vi "Construct.vi"(5 "Mailserver":string, 6 "Buffer":u32, 7 "Subject":string, 8 "Error in (no error)":errorcluster, 9 "Recipients":string[](array[string]), 10 "LogFormatterInterface in":refnum<class "LogFormatterInterface.lvclass">) -> (0 "Error out":errorcluster, 3 "LogWriterEmail out":refnum<class "LogWriterEmail.lvclass">)   [LabVIEW 2011, in "LogWriterEmail.lvclass"]
uses:
  LogWriterEmail.lvclass
  Formatter/LogFormatterInterface/LogFormatterInterface.lvclass
  LogWriterEmail.lvclass/LogWriterEmail.ctl
  LogWriterMock/LogWriterMock.lvclass
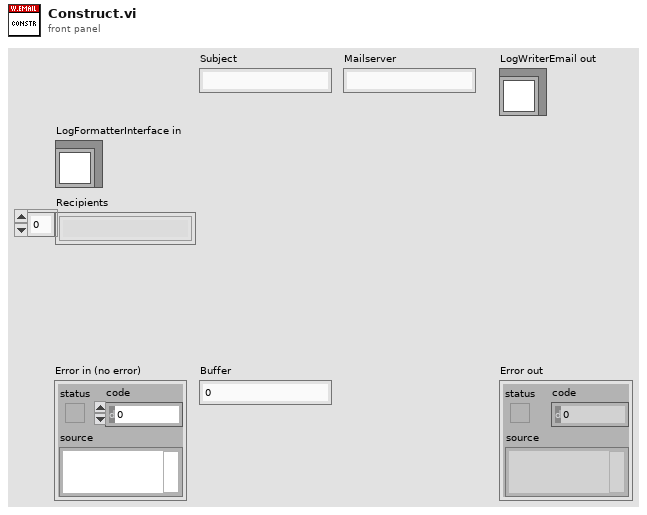
[diagram p1: front panel]
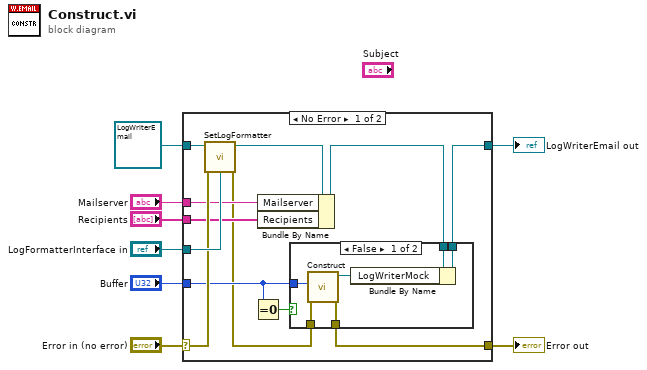
[diagram p0: block diagram]
diagram:
  n1 = case shown="No Error" "Error in (no error)" {
    selector: "Error in (no error)" -> [w18 w30]
    tunnel: [w11 w30] -> w7
    tunnel: [w9 w29] -> w6
    tunnel: refnum<class "LogWriterEmail.lvclass"> refnum ("LogWriterEmail in") -> [w19 w29]
    tunnel: "LogFormatterInterface in" -> [w20 _]
    tunnel: "Mailserver" -> [w16 _]
    tunnel: "Recipients" -> [w15 _]
    tunnel: "Buffer" -> [w13 _]
    frame No Error {
      n2 = call-dynamic "SetLogFormatter.vi"("Error in (no error)"=w18, "LogFormatterInterface in"=w20, "LogWriterEmail in"=w19) -> ("Error out"=w12:errorcluster, "LogWriterEmail out"=w17:refnum<class "LogWriterEmail.lvclass">)  [unwired: 7 in]
      n3 = Equal To 0?(x=w13) -> (x = 0?=w14:bool)
      n4 = Bundle By Name(cluster=w17, "Mailserver"=w16, "Recipients"=w15) -> (w10:refnum<class "LogWriterEmail.lvclass">)
      n5 = case shown="False" w14 {
        tunnel: w13 -> [w26 _]
        tunnel: w10 -> [w22 w28]
        tunnel: w12 -> [w25 w27]
        tunnel: [w24 w27] -> w11
        tunnel: [w21 w28] -> w9
        frame False {
          n6 = call "Construct.vi"("Error in (no error)"=w25, "Buffer"=w26) -> ("Error out"=w24:errorcluster, "LogWriterMock out"=w23:refnum<class "LogWriterMock.lvclass">)  [unwired: 8 in]
          n7 = Bundle By Name(cluster=w22, "LogWriterMock"=w23) -> (w21:refnum<class "LogWriterEmail.lvclass">)
        }
        frame True {
        }
      }
    }
    frame Error {
    }
  }
  "Error out" <- w7
  "LogWriterEmail out" <- w6
